vi "Frame to Image Data.vi"(8 "error in (no error)":errorcluster, 11 "Frame":string) -> (0 "error out":errorcluster, 3 "Image Data":T1)   [LabVIEW 2015, in "MJPEG Reader.lvclass"]
doc: "Convert JPEG image data into a LabVIEW Image Data format."
uses:
  MJPEG Reader.lvclass
  <vilib>/picture/picture.llb/imagedata.ctl
  System.Drawing
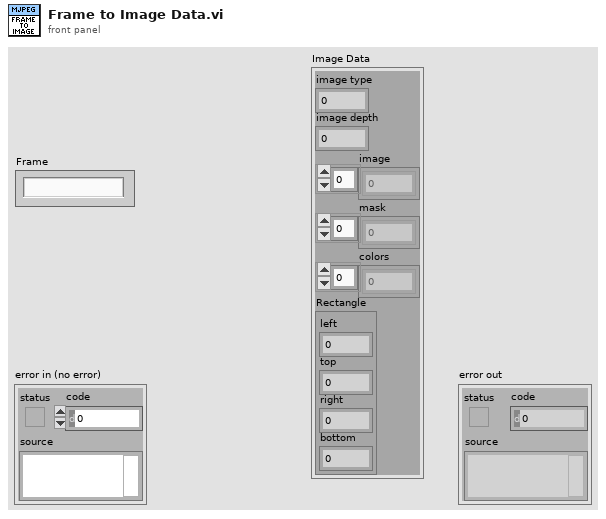
[diagram p1: front panel]
types:
  T1 = typedef "imagedata.ctl" = cluster{"image type":i32, "image depth":i32, "image":u8[], "mask":u8[], "colors":u32[], "Rectangle":cluster{"left":i16, "top":i16, "right":i16, "bottom":i16}}
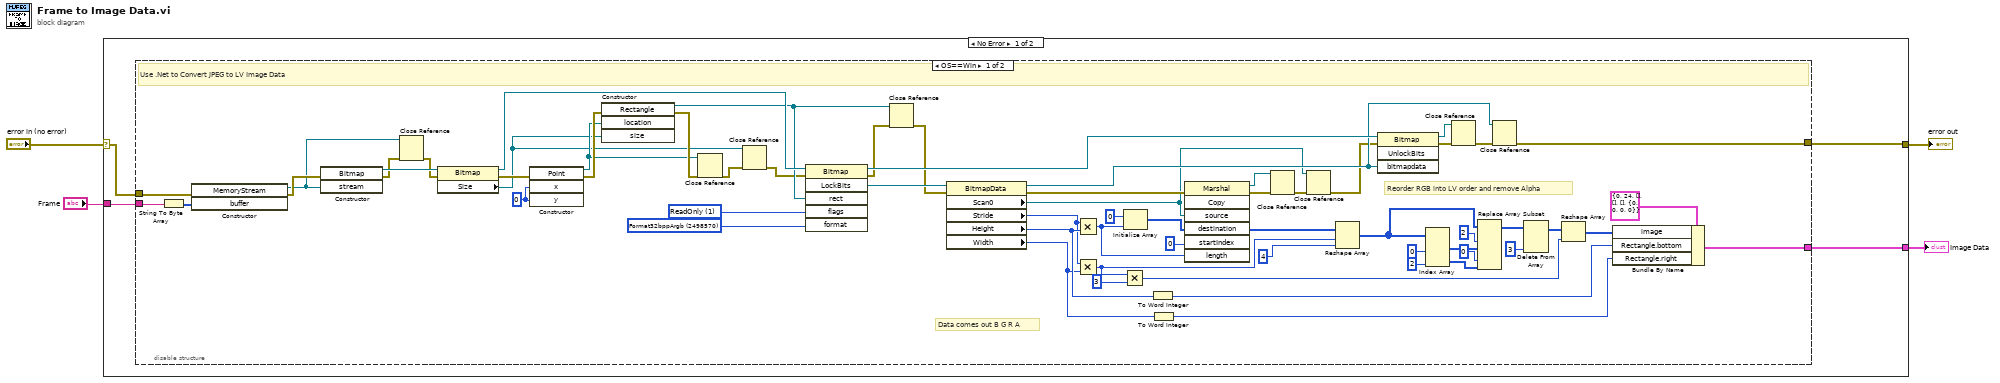
[diagram p0: block diagram]
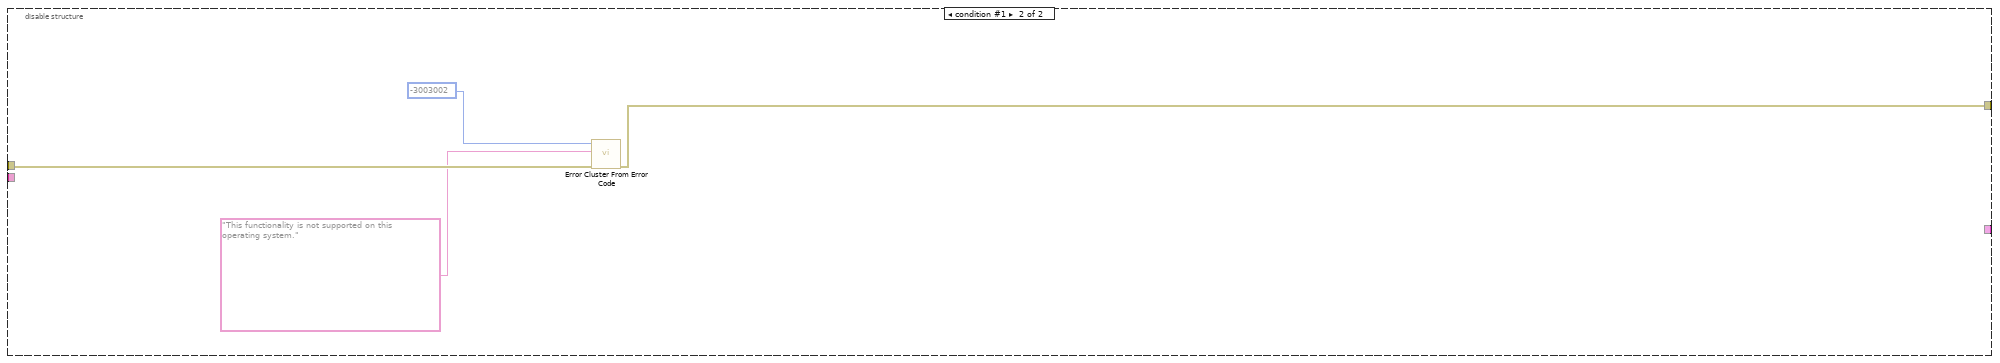
[diagram p2: hidden frame]
diagram:
  n1 = case shown="No Error" "error in (no error)" {
    selector: "error in (no error)" -> [w7 w75]
    tunnel: [w6 w75] -> w3
    tunnel: "Frame" -> [w8 _]
    tunnel: [w5 _] -> w1
    frame No Error {
      n2 = disable-structure shown="OS==Win" {
        disable-tunnel: w8 -> [w32 _]
        disable-tunnel: w7 -> [w31 w74]
        disable-tunnel: [w12 w71] -> w6
        disable-tunnel: [w18 _] -> w5
        frame condition #0 (active) {
          w36 = 0 ("x")
          w62 = 2498570 items=["DontCare, Undefined"=0, "Max"=15, "Indexed"=65536, "Gdi"=131072, "Format16bppRgb555"=135173, "Format16bppRgb565"=135174, "Format24bppRgb"=137224, "Format32bppRgb"=139273, "Format1bppIndexed"=196865, "Format4bppIndexed"=197634, "Format8bppIndexed"=198659, "Alpha"=262144, "Format16bppArgb1555"=397319, "PAlpha"=524288, "Format32bppPArgb"=925707, "Extended"=1048576, "Format16bppGrayScale"=1052676, "Format48bppRgb"=1060876, "Format64bppPArgb"=1851406, "Canonical"=2097152, "Format32bppArgb"=2498570, "Format64bppArgb"=3424269] ("format")
          w70 = 1 items=["ReadOnly"=1, "WriteOnly"=2, "ReadWrite"=3, "UserInputBuffer"=4] ("flags")
          # "Data comes out B G R A"
          # "Reorder RGB into LV order and remove Alpha"
          # "Use .Net to Convert JPEG to LV Image Data"
          n3 = String To Byte Array(string=w32) -> (unsigned byte array=w33:u8[])
          n4 = constructor class="MemoryStream"(error in=w31, "buffer"=w33) -> (reference out=w28:refnum<k24>, error out=w39:errorcluster)  [unwired: 2 in, 2 out]
          n5 = constructor class="Bitmap"(error in=w39, "stream"=w28) -> (reference out=w37:refnum<k24>, error out=w29:errorcluster)  [unwired: 2 in, 2 out]
          n6 = Close Reference(reference=w28, error in (no error)=w29) -> (error out=w30:errorcluster)
          n7 = property class="Bitmap"(reference=w37, error in=w30) -> (reference out=w38:refnum<k24>, error out=w35:errorcluster, "Size"=w16:refnum<k24>)
          n8 = constructor class="Point"(error in=w35, "x"=w36, "y"=w36) -> (reference out=w26:refnum<k24>, error out=w34:errorcluster)  [unwired: 2 in, 3 out]
          n9 = constructor class="Rectangle"(error in=w34, "location"=w26, "size"=w16) -> (reference out=w24:refnum<k24>, error out=w27:errorcluster)  [unwired: 2 in, 3 out]
          n10 = Close Reference(reference=w26, error in (no error)=w27) -> (error out=w17:errorcluster)
          n11 = Close Reference(reference=w16, error in (no error)=w17) -> (error out=w15:errorcluster)
          n12 = invoke class="Bitmap" method="LockBits"(reference=w38, error in=w15, "rect"=w24, "flags"=w70, "format"=w62) -> (reference out=w63:refnum<k24>, error out=w25:errorcluster, "LockBits"=w64:refnum<k24>)  [unwired: 1 in, 3 out]
          n13 = Close Reference(reference=w24, error in (no error)=w25) -> (error out=w23:errorcluster)
          n14 = property class="BitmapData"(reference=w64, error in=w23) -> (reference out=w13:refnum<k24>, error out=w69:errorcluster, "Scan0"=w9:refnum<k24>, "Stride"=w56:i32, "Height"=w58:i32, "Width"=w55:i32)
          n15 = Multiply(x=w56, y=w58) -> (x*y=w57:i32)
          n16 = Multiply(x=w56, y=w55) -> (x*y=w54:i32)
          n17 = Multiply(x=w54, y=3) -> (x*y=w43:i32)
          n18 = Initialize Array(u8 0, w57) -> (w67:u8[])
          n19 = To Word Integer(number=w58) -> (16bit integer=w60:i16)
          n20 = To Word Integer(number=w55) -> (16bit integer=w59:i16)
          n21 = invoke class="Marshal" method="Copy"(error in=w69, "source"=w9, "destination"=w67, "startIndex"=0, "length"=w57) -> (reference out=w22:refnum<k24>, error out=w65:errorcluster, "destination"=w53:u8[])  [unwired: 2 in, 4 out]
          n22 = Close Reference(reference=w22, error in (no error)=w65) -> (error out=w11:errorcluster)
          n23 = Close Reference(reference=w9, error in (no error)=w11) -> (error out=w10:errorcluster)
          n24 = Reshape Array(w53, w54, 4) -> (w19:u8[][])
          n25 = invoke class="Bitmap" method="UnlockBits"(reference=w63, error in=w10, "bitmapdata"=w13) -> (reference out=w20:refnum<k24>, error out=w21:errorcluster)  [unwired: 1 in, 2 out]
          n26 = Index Array(array=w19, index (col) #1=0 ("disabled index (col)"), index (col) #2=2 ("index (col)")) -> (element #1=w48:u8[], element #2=w46:u8[])  [unwired: 2 in]
          n27 = Close Reference(reference=w20, error in (no error)=w21) -> (error out=w14:errorcluster)
          n28 = Replace Array Subset(array=w19, new element #1=w48, index (col) #1=2 ("disabled index (col)"), new element #2=w46, index (col) #2=0 ("index (col)")) -> (w44:u8[][])  [unwired: 2 in]
          n29 = Close Reference(reference=w13, error in (no error)=w14) -> (error out=w12:errorcluster)
          n30 = Delete From Array(array=w44, index (col)=3 ("disabled index (col)")) -> (array with subset deleted=w41:u8[][])  [unwired: 2 in, 1 out]
          n31 = Reshape Array(w41, w43) -> (w42:u8[])
          n32 = Bundle By Name(cluster=T1 {"image type"=0, "image depth"=24, "image"=[], "mask"=[], "colors"=[], "Rectangle"={"left"=0, "top"=0, "right"=0, "bottom"=0}} ("image data"), "image"=w42, "Rectangle.bottom"=w60, "Rectangle.right"=w59) -> (w18:T1)
        }
        frame condition #1 {
          n33 = call <vilib>:"Error Cluster From Error Code.vi"("error in (no error)"=w74, "error message (\"\")"="This functionality is not supported on this operating system." ("error message (\"\")"), "error code (0)"=-3003002) -> ("error out"=w71:errorcluster)  [unwired: 6 in]
        }
      }
    }
    frame Error {
    }
  }
  "error out" <- w3
  "Image Data" <- w1
